vi "Stop Core.vi"(10 "final error code":i32, 11 "CS++Fgen in":refnum<class "CS++Fgen.lvclass">) -> (3 "CS++Fgen out":refnum<class "CS++Fgen.lvclass">)   [LabVIEW 2013, in "CS++Fgen.lvlib" / "CS++Fgen.lvclass"]
doc: "(<B>Filename</B>: Actor Framework.lvlib:Actor.lvclass:Stop Core.vi)\n\nDefines what the actor does before it stops. Use the <B>final error code</B> input to determine whether the actor shut down in response to an error.\n\nBy default, this method does nothing. A descendant class may override it to define behavior, such as shutting down any processes the actor initiated in its override of the Actor Core method."
uses:
  CS++Fgen.lvclass
  <vilib>/ActorFramework/Time-Delayed Send Message/Time-Delay Override Options.ctl
  CSPP_Core/Actors/CS++DeviceActor/CS++DeviceActor.lvclass
  CS++Fgen.lvclass/CS++Fgen.ctl
  CSPP_Core/Classes/CS++ProcessVariables/PVConnection/PVConnection.lvclass
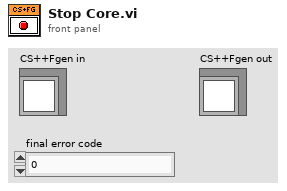
[diagram p1: front panel]
types:
  T1 = typedef "Time-Delay Override Options.ctl" = enum16{"Send next copy now", "Skip next scheduled copy", "Send next copy now and stop all further copies", "Stop all further copies"}
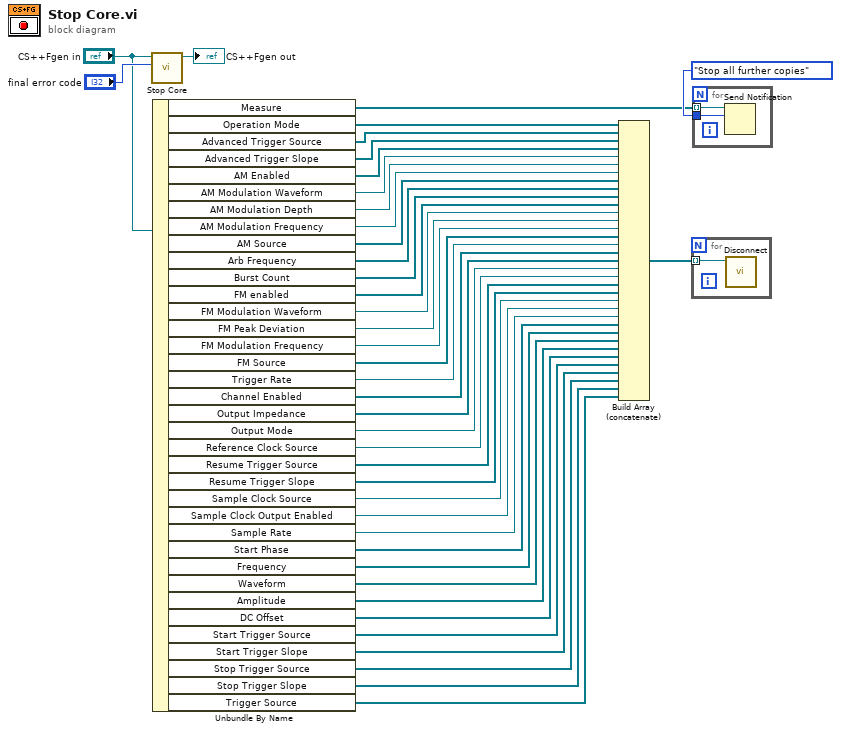
[diagram p0: block diagram]
diagram:
  n1 = call-parent "Stop Core.vi"("final error code"="final error code", "CS++DeviceActor in"="CS++Fgen in") -> ("CS++DeviceActor out"=→"CS++Fgen out":refnum<class "CS++Fgen.lvclass">)  [unwired: 9 in]
  n2 = Unbundle By Name("CS++Fgen in") -> ("Measure"=w36:refnum<notifier>[], "Operation Mode"=w35:refnum<class "PVConnection.lvclass">[], "Advanced Trigger Source"=w34:refnum<class "PVConnection.lvclass">[], "Advanced Trigger Slope"=w33:refnum<class "PVConnection.lvclass">[], "AM Enabled"=w32:refnum<class "PVConnection.lvclass">[], "AM Modulation Waveform"=w31:refnum<class "PVConnection.lvclass">, "AM Modulation Depth"=w30:refnum<class "PVConnection.lvclass">, "AM Modulation Frequency"=w29:refnum<class "PVConnection.lvclass">, "AM Source"=w28:refnum<class "PVConnection.lvclass">[], "Arb Frequency"=w27:refnum<class "PVConnection.lvclass">[], "Burst Count"=w26:refnum<class "PVConnection.lvclass">[], "FM enabled"=w25:refnum<class "PVConnection.lvclass">[], "FM Modulation Waveform"=w24:refnum<class "PVConnection.lvclass">, "FM Peak Deviation"=w23:refnum<class "PVConnection.lvclass">, "FM Modulation Frequency"=w22:refnum<class "PVConnection.lvclass">, "FM Source"=w21:refnum<class "PVConnection.lvclass">[], "Trigger Rate"=w20:refnum<class "PVConnection.lvclass">, "Channel Enabled"=w19:refnum<class "PVConnection.lvclass">[], "Output Impedance"=w18:refnum<class "PVConnection.lvclass">[], "Output Mode"=w17:refnum<class "PVConnection.lvclass">, "Reference Clock Source"=w16:refnum<class "PVConnection.lvclass">, "Resume Trigger Source"=w15:refnum<class "PVConnection.lvclass">[], "Resume Trigger Slope"=w14:refnum<class "PVConnection.lvclass">[], "Sample Clock Source"=w13:refnum<class "PVConnection.lvclass">, "Sample Clock Output Enabled"=w12:refnum<class "PVConnection.lvclass">, "Sample Rate"=w11:refnum<class "PVConnection.lvclass">, "Start Phase"=w10:refnum<class "PVConnection.lvclass">[], "Frequency"=w9:refnum<class "PVConnection.lvclass">[], "Waveform"=w8:refnum<class "PVConnection.lvclass">[], "Amplitude"=w7:refnum<class "PVConnection.lvclass">[], "DC Offset"=w6:refnum<class "PVConnection.lvclass">[], "Start Trigger Source"=w5:refnum<class "PVConnection.lvclass">[], "Start Trigger Slope"=w4:refnum<class "PVConnection.lvclass">[], "Stop Trigger Source"=w3:refnum<class "PVConnection.lvclass">[], "Stop Trigger Slope"=w2:refnum<class "PVConnection.lvclass">[], "Trigger Source"=w1:refnum<class "PVConnection.lvclass">[])
  n3 = Build Array (concatenate)(w35, w34, w33, w32, w31, w30, w29, w28, w27, w26, w25, w24, w23, w22, w21, w20, w19, w18, w17, w16, w15, w14, w13, w12, w11, w10, w9, w8, w7, w6, w5, w4, w3, w2, w1) -> (w38:refnum<class "PVConnection.lvclass">[])
  n4 = for {
    tunnel: w38 -> [w42] mode=indexing
    n5 = call-dynamic "Disconnect.vi"("PVConnection in"=w42) -> ()  [unwired: 9 in, 2 out]
  }
  n6 = for {
    tunnel: w36 -> [w44] mode=indexing
    tunnel: Time-Delay_Override_Options."Stop all further copies" ("notification") -> [w43]
    n7 = Send Notification(notification=w43, notifier=w44) -> ()  [unwired: 1 in, 2 out]
  }
